vi "DWF FGEN Configure Arbitrary Waveform.vi"(0 "Instrument Handle In":u32, 7 "Waveform":waveform(dbl), 11 "Error In":errorcluster caption="Error In (no error)") -> (4 "Instrument Handle Out":u32, 15 "Error Out":errorcluster)   [LabVIEW 2015, in "DigilentWF.lvlib"]
doc: "Configures the instrument to output a waveform. The waveform is output either after the end of the current waveform if output is enabled, or immediately after output is enabled. Any unwired configuration terminals do not change the existing values of those parameters."
uses:
  <vilib>/DigilentWF/DigilentWF.lvlib
  dwf.dll
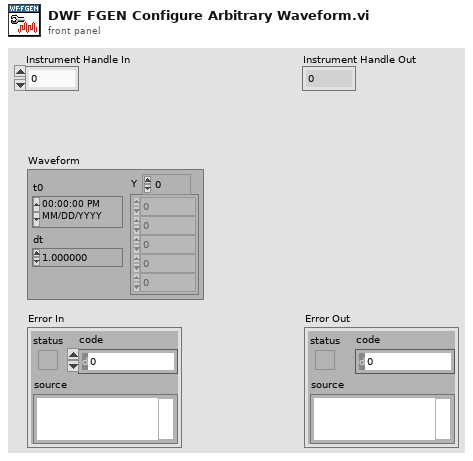
[diagram p1: front panel]
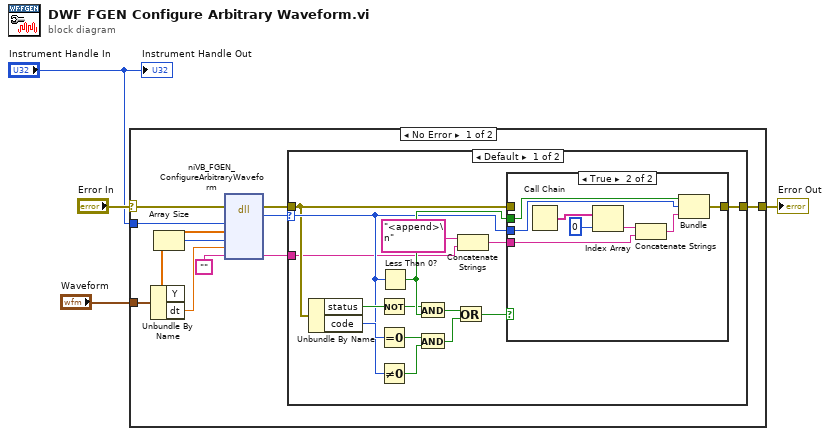
[diagram p0: block diagram]
diagram:
  n1 = case "outter_case" shown="No Error" "Error In" {
    selector: "Error In" -> [w13 w41]
    tunnel: [w15 w41] -> w3
    tunnel: "Instrument Handle In" -> [w10 _]
    tunnel: "Waveform" -> [w14 _]
    frame No Error {
      n2 = Unbundle By Name(w14) -> ("Y"=w9:dbl[], "dt"=w7:dbl)
      n3 = Array Size(array=w9) -> (size(s)=w8:i32)
      n4 = dll-call lib="dwf.*" fn="niVB_FGEN_ConfigureArbitraryWaveform"(error in=w13, "instrumentHandle"=w10, "waveform"=w9, "waveformSize"=w8, "samplePeriod"=w7, "szError"="") -> (error out=w12:errorcluster, "return type"=w11:i32, "szError"=w5:string)  [unwired: 6 in, 1 out]
      n5 = case "inner_case" shown="Default" w11 {
        selector: w11 -> [w21 _]
        tunnel: w12 -> [w17 w40]
        tunnel: [w18 w40] -> w15
        tunnel: w5 -> [w16 _]
        frame Default {
          n6 = Unbundle By Name(w17) -> ("status"=w25:bool, "code"=w29:i32)
          n7 = Not(x=w25) -> (.not. x?=w28:bool)
          n8 = Equal To 0?(x=w29) -> (x = 0?=w24:bool)
          n9 = Not Equal To 0?(x=w21) -> (x != 0?=w27:bool)
          n10 = Less Than 0?(x=w21) -> (x < 0?=w30:bool)
          n11 = And(x=w28, y=w30) -> (x .and. y?=w26:bool)
          n12 = And(x=w24, y=w27) -> (x .and. y?=w23:bool)
          n13 = Or(x=w26, y=w23) -> (x .or. y?=w22:bool)
          n14 = Concatenate Strings("<append>\n" ("string"), w16) -> (w20:string)
          n15 = case shown="True" w22 {
            tunnel: [w31 w38] -> w18
            tunnel: w21 -> [_ w37]
            tunnel: w30 -> [_ w36]
            tunnel: w17 -> [w31 _]
            tunnel: w20 -> [_ w32]
            frame False {
            }
            frame True {
              n16 = Call Chain() -> (call chain=w35:string[])
              n17 = Index Array(array=w35, index=0) -> (element=w34:string)
              n18 = Concatenate Strings(w34, w32) -> (w39:string)
              n19 = Bundle(w36, "return type"=w37, w39) -> (w38:cluster{bool, "return type":i32, string})  [unwired: 1 out]
            }
          }
        }
        frame 0 {
        }
      }
    }
    frame Error {
    }
  }
  "Error Out" <- w3
  "Instrument Handle Out" <- "Instrument Handle In"
